vi "Cursor Positions Write.vi"(4 "error in (no error)":errorcluster, 5 "Value":cluster{"Left":dbl, "Right":dbl}, 6 "Container State":T4, 7 "Display State In":T1={"Numeric"=0.0, "Timeline Ref"=refnum, "Waveform Ref"=refnum, "Fill Plots"=FALSE, "Cursor Redraw"=TRUE}) -> (0 "error out":errorcluster, 3 "Display State Out":T1={"Numeric"=0.0, "Timeline Ref"=refnum, "Waveform Ref"=refnum, "Fill Plots"=FALSE, "Cursor Redraw"=TRUE})   [LabVIEW 2017, in "XGrapher.xctl"]
doc: "Stops waveform graph from redrawing during cursor movement. Set this to false if graph performance is slow due to large data sets"
uses:
  XGrapher.xctl
  <vilib>/_xctls/Container State.ctl
  State 1.ctl
  Typedefs/Xctrl-Timeline graph ref.ctl
  Typedefs/Xctrl-Waveform graph ref.ctl
  <vilib>/_xctls/XControlSupport.lvlib
panel:
  # "Replace the Value Control below with a Control of desired type.\nDo not remove this Control or the others from the connector pane.\nDo not change the connector pane pattern.\nThe Value control should always be the third terminal from top on the input side in the connector pane."
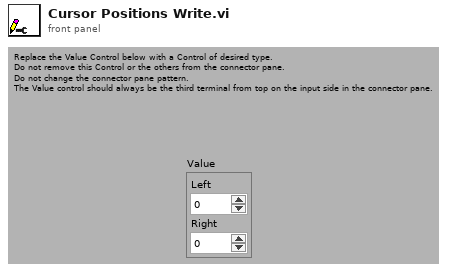
[diagram p1: front panel]
types:
  T1 = typedef "XGrapher.xctl/State 1.ctl" = cluster{"Numeric":dbl, "Timeline Ref":T2, "Waveform Ref":T3, "Fill Plots":bool, "Cursor Redraw":bool}
  T2 = typedef "XGrapher.xctl/Xctrl-Timeline graph ref.ctl" = refnum<vi>
  T3 = typedef "XGrapher.xctl/Xctrl-Waveform graph ref.ctl" = refnum<vi>
  T4 = typedef "XControlSupport.lvlib/Container State.ctl" = cluster{"Indicator?":bool, "Run Mode?":bool, " Refnum":refnum<vi>}
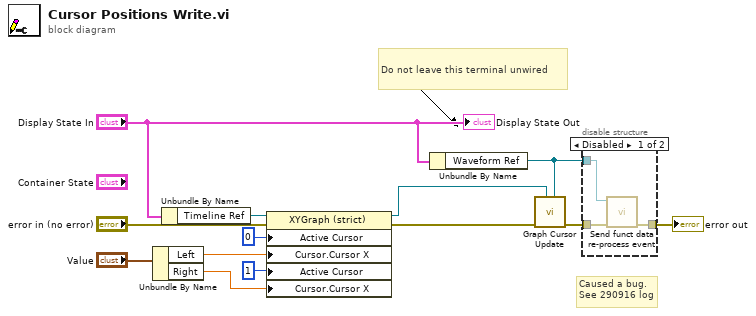
[diagram p0: block diagram]
diagram:
  # "Caused a bug.\nSee 290916 log"
  # "Do not leave this terminal unwired"
  n1 = Unbundle By Name("Value") -> ("Left"=w10:dbl, "Right"=w5:dbl)
  n2 = Unbundle By Name("Display State In") -> ("Timeline Ref"=w7:T2)
  n3 = property on="Property Node" class="XYGraph (strict)"(reference=w7, error in="error in (no error)", "Active Cursor"=u32 0, "Cursor.Cursor X"=w10, "Active Cursor"=u32 1, "Cursor.Cursor X"=w5) -> (reference out=w6:T2, error out=w8:errorcluster)
  n4 = Unbundle By Name("Display State In") -> ("Waveform Ref"=w1:T3)
  n5 = call "Graph Cursor Update.vi"("Waveform Ref in"=w1, "Timeline Ref in"=w6, "error in (no error)"=w8) -> ("error out"=w3:errorcluster)  [unwired: 6 in, 2 out]
  n6 = disable-structure shown="Disabled" {
    disable-tunnel: w3 -> [w16 w17]
    disable-tunnel: [w15 w17] -> w2
    disable-tunnel: w1 -> [w14 _]
    frame Disabled {
      n7 = call "Send funct data re-process event.vi"("error in (no error)"=w16, "Waveform Graph in"=w14) -> ("error out"=w15:errorcluster)  [unwired: 9 in]
    }
    frame Enabled {
    }
  }
  "error out" <- w2
  "Display State Out" <- "Display State In"
